vi "two counters test.vi"() -> ()   [LabVIEW 2012, in "Waveform.lvclass"]
uses:
  Waveform.lvclass
  <vilib>/DAQmx/write.llb/DAQmx Write (Digital Wfm 1Chan NSamp).vi
  <vilib>/DAQmx/create/channels.llb/DAQmx Create Channel (DO-Digital Output).vi
  <vilib>/Waveform/DWDTOps.llb/Digital Pattern Generator (Ramp).vi
  <vilib>/DAQmx/configure/events/hardwareSignals.llb/DAQmx Export Signal (Most Signals).vi
  <vilib>/DAQmx/create/channels.llb/DAQmx Create Channel (CO-Pulse Generation-Frequency).vi
  <vilib>/DAQmx/configure/timing.llb/DAQmx Timing (Implicit).vi
  <vilib>/DAQmx/configure/trigger.llb/DAQmx Start Trigger (Digital Edge).vi
  <vilib>/Waveform/DWDTOps.llb/DWDT Uncompress Digital.vi
  <vilib>/DAQmx/miscellaneous.llb/DAQmx Fill In Error Info.vi
  <resource>/objmgr/daqmx.rc
panel:
  in  "C1 initial delay (s)":dbl format="%.6f"
  in  "C2 duty cycle":dbl=0.5 format="%.6f"
  in  "C1 duty cycle":dbl=0.5 format="%.6f"
  out "error out":errorcluster
  in  "Boolean":bool
  in  "C2 frequency":dbl=1.0 format="%.6f"
  in  "C1 frequency":dbl=1.0 format="%.6f"
  in  "error in":errorcluster
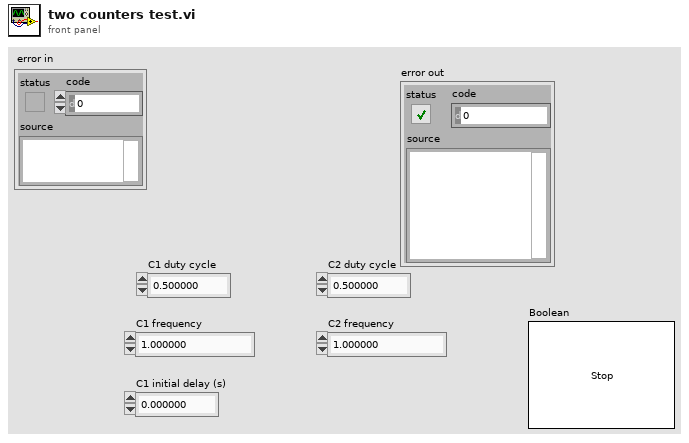
[diagram p1: front panel]
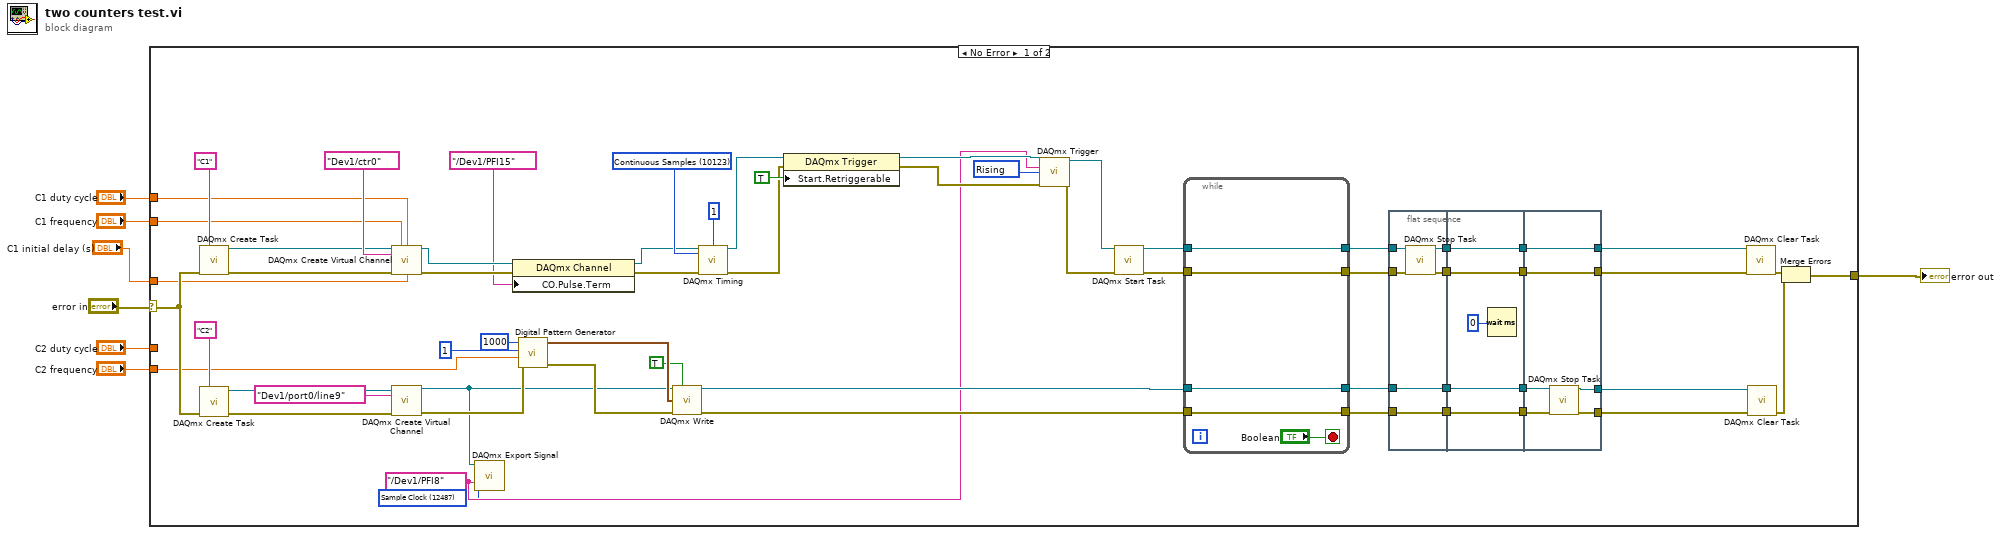
[diagram p0: block diagram]
diagram:
  n1 = case shown="No Error" "error in" {
    selector: "error in" -> [w58 w90]
    tunnel: "C1 frequency" -> [w59 _]
    tunnel: "C2 frequency" -> [w22 _]
    tunnel: [w48 w90] -> w4
    tunnel: "C1 duty cycle" -> [w45 _]
    tunnel: "C2 duty cycle" -> [_ _]
    tunnel: "C1 initial delay (s)" -> [w43 _]
    frame No Error {
      w8 = 12487 items=["AI Convert Clock"=12484, "10MHz Reference Clock"=12536, "20MHz Timebase Clock"=12486, "Sample Clock"=12487, "Advance Trigger"=12488, "Reference Trigger"=12490, "Start Trigger"=12491, "Advance Complete Event"=12492, "AI Hold Complete Event"=12493, "Counter Output Event"=12494, "Change Detection Event"=12511, "Watchdog Timer Expired Event"=12512] ("signal")
      w9 = tag "/Dev1/PFI8" ("output terminal")
      w40 = 10280 items=["Rising"=10280, "Falling"=10171] ("edge")
      w56 = 10123 items=["Finite Samples"=10178, "Continuous Samples"=10123, "Hardware Timed Single Point"=12522] ("sample mode")
      n2 = call <vilib>:"DAQmx Create Task.vi"("new task name"="C1", "error in"=w58) -> ("task out"=w42:refnum<k21>, "error out"=w65:errorcluster)  [unwired: 12 in]
      n3 = call <vilib>:"DAQmx Create Task.vi"("new task name"="C2", "error in"=w58) -> ("task out"=w63:refnum<k21>, "error out"=w62:errorcluster)  [unwired: 12 in]
      n4 = call-poly <vilib>:"DAQmx Create Virtual Channel.vi"("task in"=w42, "frequency"=w59, "duty cycle"=w45, "counter"=tag "Dev1/ctr0", "error in"=w65, "initial delay"=w43) -> ("task out"=w60:refnum<k21>, "error out"=w61:errorcluster)  [unwired: 8 in]
      n5 = call-poly <vilib>:"DAQmx Create Virtual Channel.vi"("task in"=w63, "lines"=tag "Dev1/port0/line9", "error in"=w62) -> ("task out"=w10:refnum<k21>, "error out"=w26:errorcluster)  [unwired: 11 in]
      n6 = call-poly <vilib>:"DAQmx Export Signal.vi"("task/channels in"=w10, "signal"=w8, "output terminal"=w9) -> ()  [unwired: 11 in, 2 out]
      n7 = property class="DAQmx Channel"(reference=w60, error in=w61, "CO.Pulse.Term"=tag "/Dev1/PFI15") -> (reference out=w55:refnum<k21>, error out=w57:errorcluster)
      n8 = call-poly <vilib>:"Digital Pattern Generator.vi"("error in (no error)"=w26, "sample rate"=w22, "number of signals"=u32 1, "number of samples"=u32 1000) -> ("error out"=w25:errorcluster, "digital waveform"=w21:digitalwaveform)  [unwired: 6 in]
      n9 = call-poly <vilib>:"DAQmx Write.vi"("task/channels in"=w10, "auto start"=TRUE, "data"=w21, "error in"=w25) -> ("task out"=w17:refnum<k21>, "error out"=w19:errorcluster)  [unwired: 9 in, 1 out]
      n10 = call-poly <vilib>:"DAQmx Timing.vi"("task/channels in"=w55, "sample mode"=w56, "samples per channel"=1, "error in"=w57) -> ("task out"=w16:refnum<k21>, "error out"=w13:errorcluster)  [unwired: 10 in]
      n11 = property class="DAQmx Trigger"(reference=w16, error in=w13, "Start.Retriggerable"=TRUE) -> (reference out=w18:refnum<k21>, error out=w14:errorcluster)
      n12 = call-poly <vilib>:"DAQmx Trigger.vi"("task/channels in"=w18, "source"=w9, "edge"=w40, "error in"=w14) -> ("task out"=w15:refnum<k21>, "error out"=w12:errorcluster)  [unwired: 10 in]
      n13 = call <vilib>:"DAQmx Start Task.vi"("task/channels in"=w15, "error in"=w12) -> ("task out"=w47:refnum<k21>, "error out"=w52:errorcluster)  [unwired: 12 in]
      n14 = while {
        tunnel: w19 -> [w88]
        tunnel: [w88] -> w30
        tunnel: w52 -> [w87]
        tunnel: [w87] -> w51
        tunnel: w47 -> [w86]
        tunnel: [w86] -> w46
        tunnel: w17 -> [w85]
        tunnel: [w85] -> w36
        stop <- "Boolean" stop-if-true
      }
      n15 = flat-sequence {
        tunnel: w51 -> [w71]
        tunnel: w46 -> [w70]
        tunnel: [w73] -> w39
        tunnel: [w72] -> w38
        tunnel: [w69] -> w37
        tunnel: w36 -> [w69]
        tunnel: [w68] -> w31
        tunnel: w30 -> [w68]
        tunnel: w39 -> [w78]
        tunnel: w38 -> [w77]
        tunnel: w37 -> [w75]
        tunnel: [w78] -> w35
        tunnel: [w77] -> w34
        tunnel: [w75] -> w33
        tunnel: [w74] -> w32
        tunnel: w31 -> [w74]
        tunnel: [w83] -> w53
        tunnel: [w84] -> w54
        tunnel: w35 -> [w84]
        tunnel: w34 -> [w83]
        tunnel: w33 -> [w81]
        tunnel: w32 -> [w82]
        tunnel: [w80] -> w29
        tunnel: [w79] -> w28
        frame #0 {
          n16 = call <vilib>:"DAQmx Stop Task.vi"("task/channels in"=w70, "error in"=w71) -> ("task out"=w73:refnum<k21>, "error out"=w72:errorcluster)  [unwired: 12 in]
        }
        frame #1 {
          n17 = Wait (ms)(milliseconds to wait=u32 0) -> ()  [unwired: 1 out]
        }
        frame #2 {
          n18 = call <vilib>:"DAQmx Stop Task.vi"("task/channels in"=w81, "error in"=w82) -> ("task out"=w80:refnum<k21>, "error out"=w79:errorcluster)  [unwired: 12 in]
        }
      }
      n19 = call <vilib>:"DAQmx Clear Task.vi"("task in"=w54, "error in"=w53) -> ("error out"=w50:errorcluster)  [unwired: 13 in]
      n20 = call <vilib>:"DAQmx Clear Task.vi"("task in"=w29, "error in"=w28) -> ("error out"=w49:errorcluster)  [unwired: 13 in]
      n21 = Merge Errors(w50, w49) -> (w48:errorcluster)
    }
    frame Error {
    }
  }
  "error out" <- w4
